vi "PT Module Tags.vi"(11 "PT Module Config":T1[](array[typedef])) -> (2 "PT Tags Array":T4[](array[typedef]), 3 "All  Numeric Tags":string[](array[string]))   [LabVIEW 2018, in "PT Module.lvlib"]
uses:
  PT Module.lvlib
  Controls/PT Module Tag Names.ctl
  Controls/PT Module Config Cluster.ctl
  <vilib>/Utility/miscctls.llb/LVPoint32TypeDef.ctl
  Tag VIs/Numeric Alarm Settings Cluster.ctl
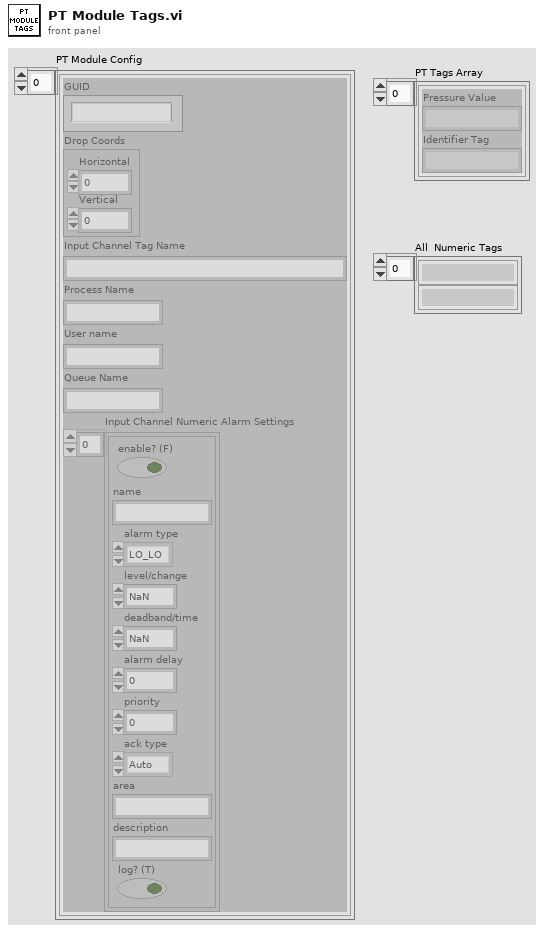
[diagram p1: front panel]
types:
  T1 = typedef "PT Module.lvlib/PT Module Config Cluster.ctl" = cluster{"GUID":string, "Drop Coords":T2, "Input Channel Tag Name ":string, "Process Name":string, "User name":string, "Queue Name":string, "Input Channel Numeric Alarm Settings":T3[]}
  T2 = typedef "LVPoint32TypeDef.ctl" = cluster{"Horizontal":i32, "Vertical":i32}
  T3 = typedef "Numeric Alarm Settings Cluster.ctl" = cluster{"enable? (F)":bool, "name":string, "alarm type":enum16{"HI_HI", "HI", "LO", "LO_LO"}, "level/change":dbl, "deadband/time":dbl, "alarm delay":dbl, "priority":u32, "ack type":enum16{"Auto", "User", "None", "Each Occurrence"}, "area":string, "description":string, "log? (T)":bool}
  T4 = typedef "PT Module.lvlib/PT Module Tag Names.ctl" = cluster{"Pressure Value":string, "Identifier Tag":string}
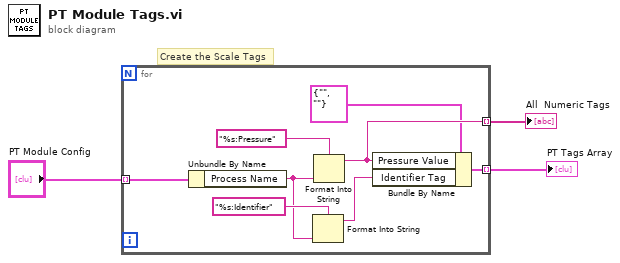
[diagram p0: block diagram]
diagram:
  # "Create the Scale Tags"
  n1 = for {
    tunnel: "PT Module Config" -> [w8] mode=indexing
    tunnel: [w9] -> w3 mode=indexing
    tunnel: [w10] -> w2 mode=indexing
    n2 = Unbundle By Name(w8) -> ("Process Name"=w6:string)
    n3 = Format Into String(format string="%s:Identifier", w6) -> (resulting string=w5:string)  [unwired: 2 in, 1 out]
    n4 = Format Into String(format string="%s:Pressure", w6) -> (resulting string=w10:string)  [unwired: 2 in, 1 out]
    n5 = Bundle By Name(cluster=T4 {"Pressure Value"="", "Identifier Tag"=""} ("PT Module Tag Names"), "Pressure Value"=w10, "Identifier Tag"=w5) -> (w9:T4)
  }
  "PT Tags Array" <- w3
  "All  Numeric Tags" <- w2
